vi "HandleObservationSync_003.vi"(8 "error in (no error)":errorcluster, 11 "S4GUI in":refnum<class "S4GUI.lvclass">) -> (0 "error out":errorcluster, 3 "S4GUI out":refnum<class "S4GUI.lvclass">)   [LabVIEW 2018, in "S4GUI.lvclass"] (continued)
          n222 = disable-structure shown="Enabled" {
            disable-tunnel: w542 -> [w576 w589]
            disable-tunnel: w541 -> [w575 w588]
            disable-tunnel: [w574 w589] -> w540
            disable-tunnel: [w573 w588] -> w539
            frame Disabled {
              n223 = call "Read WPROT.vi"("error in (no error)"=w575, "Instrument in"=w576) -> ("error out"=w579:errorcluster, "Opt_Selector.lvclass"=w580:refnum<class "Opt_Selector.lvclass">, "Instrument out"=w586:refnum<class "Instrument.lvclass">)  [unwired: 7 in]
              n224 = call-dynamic "Read State Machine.vi"("error in (no error)"=w579, "Device in"=w580) -> ("error out"=w582:errorcluster, "State Machine.lvclass"=w584:refnum<class "State Machine.lvclass">, "Device out"=w581:refnum<class "Opt_Selector.lvclass">)  [unwired: 7 in]
              n225 = call "Next State.vi"("error in (no error)"=w582, "New_State"=30, "State Machine in"=w584) -> ("error out"=w578:errorcluster, "State Machine out"=w577:refnum<class "State Machine.lvclass">)  [unwired: 7 in]
              n226 = call-dynamic "Write State Machine.vi"("error in (no error)"=w578, "State Machine.lvclass"=w577, "Device in"=w581) -> ("error out"=w585:errorcluster, "Device out"=w587:refnum<class "Opt_Selector.lvclass">)  [unwired: 7 in]
              n227 = call "Write WPROT.vi"("error in (no error)"=w585, "Opt_Selector.lvclass"=w587, "Instrument in"=w586) -> ("error out"=w573:errorcluster, "Instrument out"=w574:refnum<class "Instrument.lvclass">)  [unwired: 7 in]
            }
            frame Enabled {
              # "depois do homing no WPSEL, o homing do WPROT é feito automaticamente pelo ICS"
            }
          }
          n228 = call "Read ASEL.vi"("error in (no error)"=w539, "Instrument in"=w540) -> ("error out"=w556:errorcluster, "Opt_Selector.lvclass"=w557:refnum<class "Opt_Selector.lvclass">, "Instrument out"=w563:refnum<class "Instrument.lvclass">)  [unwired: 7 in]
          n229 = call-dynamic "Read State Machine.vi"("error in (no error)"=w556, "Device in"=w557) -> ("error out"=w559:errorcluster, "State Machine.lvclass"=w561:refnum<class "State Machine.lvclass">, "Device out"=w558:refnum<class "Opt_Selector.lvclass">)  [unwired: 7 in]
          n230 = call "Next State.vi"("error in (no error)"=w559, "New_State"=30, "State Machine in"=w561) -> ("error out"=w555:errorcluster, "State Machine out"=w554:refnum<class "State Machine.lvclass">)  [unwired: 7 in]
          n231 = call-dynamic "Write State Machine.vi"("error in (no error)"=w555, "State Machine.lvclass"=w554, "Device in"=w558) -> ("error out"=w562:errorcluster, "Device out"=w564:refnum<class "Opt_Selector.lvclass">)  [unwired: 7 in]
          n232 = Increment(x=w565) -> (x+1=w567:u32)
          n233 = call "Write ASEL.vi"("error in (no error)"=w562, "Opt_Selector.lvclass"=w564, "Instrument in"=w563) -> ("error out"=w537:errorcluster, "Instrument out"=w538:refnum<class "Instrument.lvclass">)  [unwired: 7 in]
          n234 = call "Read GMIR.vi"("error in (no error)"=w537, "Instrument in"=w538) -> ("error out"=w545:errorcluster, "Opt_Continuous.lvclass"=w546:refnum<class "Opt_Continuous.lvclass">, "Instrument out"=w552:refnum<class "Instrument.lvclass">)  [unwired: 7 in]
          n235 = call-dynamic "Read State Machine.vi"("error in (no error)"=w545, "Device in"=w546) -> ("error out"=w548:errorcluster, "State Machine.lvclass"=w550:refnum<class "State Machine.lvclass">, "Device out"=w547:refnum<class "Opt_Continuous.lvclass">)  [unwired: 7 in]
          n236 = call "Next State.vi"("error in (no error)"=w548, "New_State"=30, "State Machine in"=w550) -> ("error out"=w544:errorcluster, "State Machine out"=w543:refnum<class "State Machine.lvclass">)  [unwired: 7 in]
          n237 = call-dynamic "Write State Machine.vi"("error in (no error)"=w544, "State Machine.lvclass"=w543, "Device in"=w547) -> ("error out"=w551:errorcluster, "Device out"=w553:refnum<class "Opt_Continuous.lvclass">)  [unwired: 7 in]
          n238 = call "Write GMIR.vi"("error in (no error)"=w551, "Opt_Continuous.lvclass"=w553, "Instrument in"=w552) -> ("error out"=w536:errorcluster, "Instrument out"=w535:refnum<class "Instrument.lvclass">)  [unwired: 7 in]
          n239 = call "Write Instrument.lvclass.vi"("error in (no error)"=w536, "Instrument.lvclass"=w535, "S4ACS_GUI in"=w572) -> ("error out"=w569:errorcluster, "S4ACS_GUI out"=w568:refnum<class "S4GUI.lvclass">)  [unwired: 7 in]
          n240 = Bundle By Name(cluster=w568, "Obs_state"=w567) -> (w566:refnum<class "S4GUI.lvclass">)
        }
        frame 223 {
          # "Espera terminar o homing de WPROT,ASEL e GFOC\nantes de seguir para o próximo estado."
          n241 = call "Read Instrument.lvclass.vi"("error in (no error)"=w614, "S4ACS_GUI in"=w615) -> ("error out"=w600:errorcluster, "Instrument.lvclass"=w601:refnum<class "Instrument.lvclass">, "S4ACS_GUI out"=w609:refnum<class "S4GUI.lvclass">)  [unwired: 7 in]
          n242 = call "Read ASEL.vi"("error in (no error)"=w600, "Instrument in"=w601) -> ("error out"=w605:errorcluster, "Opt_Selector.lvclass"=w591:refnum<class "Opt_Selector.lvclass">)  [unwired: 7 in, 1 out]
          n243 = call "Read GMIR.vi"("error in (no error)"=w600, "Instrument in"=w601) -> ("error out"=w602:errorcluster, "Opt_Continuous.lvclass"=w590:refnum<class "Opt_Continuous.lvclass">)  [unwired: 7 in, 1 out]
          n244 = disable-structure shown="Enabled" {
            disable-tunnel: [w619 w625] -> w608
            disable-tunnel: w601 -> [w618 _]
            disable-tunnel: w600 -> [w617 w625]
            disable-tunnel: [w616 0 ("State")] -> w599
            frame Disabled {
              n245 = call "Read WPROT.vi"("error in (no error)"=w617, "Instrument in"=w618) -> ("error out"=w621:errorcluster, "Opt_Selector.lvclass"=w620:refnum<class "Opt_Selector.lvclass">)  [unwired: 7 in, 1 out]
              n246 = call-dynamic "Read State Machine.vi"("error in (no error)"=w621, "Device in"=w620) -> ("error out"=w622:errorcluster, "State Machine.lvclass"=w623:refnum<class "State Machine.lvclass">)  [unwired: 7 in, 1 out]
              n247 = call-dynamic "Read State.vi"("error in (no error)"=w622, "State Machine in"=w623) -> ("error out"=w619:errorcluster, "State"=w616:i32)  [unwired: 7 in, 1 out]
            }
            frame Enabled {
            }
          }
          n248 = call-dynamic "Read State Machine.vi"("error in (no error)"=w605, "Device in"=w591) -> ("error out"=w606:errorcluster, "State Machine.lvclass"=w607:refnum<class "State Machine.lvclass">)  [unwired: 7 in, 1 out]
          n249 = call-dynamic "Read State Machine.vi"("error in (no error)"=w602, "Device in"=w590) -> ("error out"=w603:errorcluster, "State Machine.lvclass"=w604:refnum<class "State Machine.lvclass">)  [unwired: 7 in, 1 out]
          n250 = Increment(x=w611) -> (x+1=w610:u32)
          n251 = call-dynamic "Read State.vi"("error in (no error)"=w606, "State Machine in"=w607) -> ("error out"=w594:errorcluster, "State"=w598:i32)  [unwired: 7 in, 1 out]
          n252 = call-dynamic "Read State.vi"("error in (no error)"=w603, "State Machine in"=w604) -> ("error out"=w593:errorcluster, "State"=w597:i32)  [unwired: 7 in, 1 out]
          n253 = Compound Arithmetic op=ADD(w599, w598, w597) -> (w596:i32)
          n254 = Equal To 0?(x=w596) -> (x = 0?=w595:bool)
          n255 = Merge Errors(w608, w594, w593) -> (w592:errorcluster)
          n256 = Select(t=w610, s=w595, f=w611) -> (s? t:f=w612:u32)
          n257 = Bundle By Name(cluster=w609, "Obs_state"=w612) -> (w613:refnum<class "S4GUI.lvclass">)
        }
        frame 224 {
          # "40 x 0.25 = 10s"
          # "40 x 0.25 = 10s"
          # "40 x 0.25 = 10s"
          # "Manda WPSEL para OFF, CALW para OFF e ASEL para OFF"
          n258 = call "Read Instrument.lvclass.vi"("error in (no error)"=w699, "S4ACS_GUI in"=w700) -> ("error out"=w685:errorcluster, "Instrument.lvclass"=w686:refnum<class "Instrument.lvclass">, "S4ACS_GUI out"=w701:refnum<class "S4GUI.lvclass">)  [unwired: 7 in]
          n259 = call "Read WPSEL.vi"("error in (no error)"=w685, "Instrument in"=w686) -> ("error out"=w681:errorcluster, "Opt_Selector.lvclass"=w680:refnum<class "Opt_Selector.lvclass">, "Instrument out"=w693:refnum<class "Instrument.lvclass">)  [unwired: 7 in]
          n260 = call "Write target.vi"("error in (no error)"=w681, "target"=80.0, "Optics in"=w680) -> ("error out"=w684:errorcluster, "Optics out"=w679:refnum<class "Opt_Selector.lvclass">)  [unwired: 7 in]
          n261 = call "Write target name.vi"("error in (no error)"=w684, "target name"="OFF", "Optics in"=w679) -> ("error out"=w677:errorcluster, "Optics out"=w678:refnum<class "Opt_Selector.lvclass">)  [unwired: 7 in]
          n262 = call-dynamic "Read State Machine.vi"("error in (no error)"=w677, "Device in"=w678) -> ("error out"=w688:errorcluster, "State Machine.lvclass"=w690:refnum<class "State Machine.lvclass">, "Device out"=w687:refnum<class "Opt_Selector.lvclass">)  [unwired: 7 in]
          n263 = call "Next State.vi"("error in (no error)"=w688, "New_State"=1, "State Machine in"=w690) -> ("error out"=w638:errorcluster, "State Machine out"=w640:refnum<class "State Machine.lvclass">)  [unwired: 7 in]
          n264 = call-dynamic "Write Timer.vi"("error in (no error)"=w638, "Timer"=u32 40, "State Machine in"=w640) -> ("error out"=w637:errorcluster, "State Machine out"=w639:refnum<class "State Machine.lvclass">)  [unwired: 7 in]
          n265 = call-dynamic "Write State Machine.vi"("error in (no error)"=w637, "State Machine.lvclass"=w639, "Device in"=w687) -> ("error out"=w692:errorcluster, "Device out"=w694:refnum<class "Opt_Selector.lvclass">)  [unwired: 7 in]
          n266 = Increment(x=w691) -> (x+1=w696:u32)
          n267 = call "Write WPSEL.vi"("error in (no error)"=w692, "Opt_Selector.lvclass"=w694, "Instrument in"=w693) -> ("error out"=w652:errorcluster, "Instrument out"=w651:refnum<class "Instrument.lvclass">)  [unwired: 7 in]
          n268 = call "Read CALW.vi"("error in (no error)"=w652, "Instrument in"=w651) -> ("error out"=w668:errorcluster, "Opt_Selector.lvclass"=w650:refnum<class "Opt_Selector.lvclass">, "Instrument out"=w648:refnum<class "Instrument.lvclass">)  [unwired: 7 in]
          n269 = call "Write target.vi"("error in (no error)"=w668, "target"=0.0, "Optics in"=w650) -> ("error out"=w671:errorcluster, "Optics out"=w667:refnum<class "Opt_Selector.lvclass">)  [unwired: 7 in]
          n270 = call "Write target name.vi"("error in (no error)"=w671, "target name"="OFF", "Optics in"=w667) -> ("error out"=w665:errorcluster, "Optics out"=w666:refnum<class "Opt_Selector.lvclass">)  [unwired: 7 in]
          n271 = call-dynamic "Read State Machine.vi"("error in (no error)"=w665, "Device in"=w666) -> ("error out"=w673:errorcluster, "State Machine.lvclass"=w675:refnum<class "State Machine.lvclass">, "Device out"=w672:refnum<class "Opt_Selector.lvclass">)  [unwired: 7 in]
          n272 = call "Next State.vi"("error in (no error)"=w673, "New_State"=1, "State Machine in"=w675) -> ("error out"=w634:errorcluster, "State Machine out"=w635:refnum<class "State Machine.lvclass">)  [unwired: 7 in]
          n273 = call-dynamic "Write Timer.vi"("error in (no error)"=w634, "Timer"=u32 40, "State Machine in"=w635) -> ("error out"=w633:errorcluster, "State Machine out"=w632:refnum<class "State Machine.lvclass">)  [unwired: 7 in]
          n274 = call-dynamic "Write State Machine.vi"("error in (no error)"=w633, "State Machine.lvclass"=w632, "Device in"=w672) -> ("error out"=w676:errorcluster, "Device out"=w649:refnum<class "Opt_Selector.lvclass">)  [unwired: 7 in]
          n275 = call "Write CALW.vi"("error in (no error)"=w676, "Opt_Selector.lvclass"=w649, "Instrument in"=w648) -> ("error out"=w647:errorcluster, "Instrument out"=w646:refnum<class "Instrument.lvclass">)  [unwired: 7 in]
          n276 = call "Read ASEL.vi"("error in (no error)"=w647, "Instrument in"=w646) -> ("error out"=w656:errorcluster, "Opt_Selector.lvclass"=w645:refnum<class "Opt_Selector.lvclass">, "Instrument out"=w643:refnum<class "Instrument.lvclass">)  [unwired: 7 in]
          n277 = call "Write target.vi"("error in (no error)"=w656, "target"=0.0, "Optics in"=w645) -> ("error out"=w659:errorcluster, "Optics out"=w655:refnum<class "Opt_Selector.lvclass">)  [unwired: 7 in]
          n278 = call "Write target name.vi"("error in (no error)"=w659, "target name"="OFF", "Optics in"=w655) -> ("error out"=w653:errorcluster, "Optics out"=w654:refnum<class "Opt_Selector.lvclass">)  [unwired: 7 in]
          n279 = call-dynamic "Read State Machine.vi"("error in (no error)"=w653, "Device in"=w654) -> ("error out"=w661:errorcluster, "State Machine.lvclass"=w663:refnum<class "State Machine.lvclass">, "Device out"=w660:refnum<class "Opt_Selector.lvclass">)  [unwired: 7 in]
          n280 = call "Next State.vi"("error in (no error)"=w661, "New_State"=1, "State Machine in"=w663) -> ("error out"=w628:errorcluster, "State Machine out"=w629:refnum<class "State Machine.lvclass">)  [unwired: 7 in]
          n281 = call-dynamic "Write Timer.vi"("error in (no error)"=w628, "Timer"=u32 40, "State Machine in"=w629) -> ("error out"=w627:errorcluster, "State Machine out"=w626:refnum<class "State Machine.lvclass">)  [unwired: 7 in]
          n282 = call-dynamic "Write State Machine.vi"("error in (no error)"=w627, "State Machine.lvclass"=w626, "Device in"=w660) -> ("error out"=w664:errorcluster, "Device out"=w644:refnum<class "Opt_Selector.lvclass">)  [unwired: 7 in]
          n283 = call "Write ASEL.vi"("error in (no error)"=w664, "Opt_Selector.lvclass"=w644, "Instrument in"=w643) -> ("error out"=w641:errorcluster, "Instrument out"=w642:refnum<class "Instrument.lvclass">)  [unwired: 7 in]
          n284 = call "Write Instrument.lvclass.vi"("error in (no error)"=w641, "Instrument.lvclass"=w642, "S4ACS_GUI in"=w701) -> ("error out"=w698:errorcluster, "S4ACS_GUI out"=w697:refnum<class "S4GUI.lvclass">)  [unwired: 7 in]
          n285 = Bundle By Name(cluster=w697, "Obs_state"=w696) -> (w695:refnum<class "S4GUI.lvclass">)
        }
        frame 225 {
          # "Espera terminar o movimento de WPSEL, ASEL e CALW para CLEAR."
          n286 = call "Read Instrument.lvclass.vi"("error in (no error)"=w730, "S4ACS_GUI in"=w731) -> ("error out"=w713:errorcluster, "Instrument.lvclass"=w714:refnum<class "Instrument.lvclass">, "S4ACS_GUI out"=w722:refnum<class "S4GUI.lvclass">)  [unwired: 7 in]
          n287 = call "Read ASEL.vi"("error in (no error)"=w713, "Instrument in"=w714) -> ("error out"=w718:errorcluster, "Opt_Selector.lvclass"=w704:refnum<class "Opt_Selector.lvclass">)  [unwired: 7 in, 1 out]
          n288 = call "Read CALW.vi"("error in (no error)"=w713, "Instrument in"=w714) -> ("error out"=w715:errorcluster, "Opt_Selector.lvclass"=w703:refnum<class "Opt_Selector.lvclass">)  [unwired: 7 in, 1 out]
          n289 = call "Read WPSEL.vi"("error in (no error)"=w713, "Instrument in"=w714) -> ("error out"=w727:errorcluster, "Opt_Selector.lvclass"=w726:refnum<class "Opt_Selector.lvclass">)  [unwired: 7 in, 1 out]
          n290 = call-dynamic "Read State Machine.vi"("error in (no error)"=w715, "Device in"=w703) -> ("error out"=w716:errorcluster, "State Machine.lvclass"=w717:refnum<class "State Machine.lvclass">)  [unwired: 7 in, 1 out]
          n291 = call-dynamic "Read State Machine.vi"("error in (no error)"=w718, "Device in"=w704) -> ("error out"=w719:errorcluster, "State Machine.lvclass"=w720:refnum<class "State Machine.lvclass">)  [unwired: 7 in, 1 out]
          n292 = call-dynamic "Read State Machine.vi"("error in (no error)"=w727, "Device in"=w726) -> ("error out"=w728:errorcluster, "State Machine.lvclass"=w729:refnum<class "State Machine.lvclass">)  [unwired: 7 in, 1 out]
          n293 = call-dynamic "Read State.vi"("error in (no error)"=w719, "State Machine in"=w720) -> ("error out"=w707:errorcluster, "State"=w711:i32)  [unwired: 7 in, 1 out]
          n294 = call-dynamic "Read State.vi"("error in (no error)"=w716, "State Machine in"=w717) -> ("error out"=w706:errorcluster, "State"=w710:i32)  [unwired: 7 in, 1 out]
          n295 = call-dynamic "Read State.vi"("error in (no error)"=w728, "State Machine in"=w729) -> ("error out"=w721:errorcluster, "State"=w712:i32)  [unwired: 7 in, 1 out]
          n296 = Compound Arithmetic op=ADD(w712, w711, w710) -> (w709:i32)
          n297 = Equal To 0?(x=w709) -> (x = 0?=w708:bool)
          n298 = Merge Errors(w721, w707, w706) -> (w705:errorcluster)
          n299 = Select(t=u32 0, s=w708, f=w723) -> (s? t:f=w724:u32)
          n300 = Bundle By Name(cluster=w722, "Obs_state"=w724) -> (w725:refnum<class "S4GUI.lvclass">)
        }
        frame 230 {
          # "PARK:\nWPSEL = OFF\n(WPROT=NA)\nCALW=SHUTTER\nASEL=OFF"
          n301 = call "Read Instrument.lvclass.vi"("error in (no error)"=w800, "S4ACS_GUI in"=w801) -> ("error out"=w793:errorcluster, "Instrument.lvclass"=w794:refnum<class "Instrument.lvclass">, "S4ACS_GUI out"=w735:refnum<class "S4GUI.lvclass">)  [unwired: 7 in]
          n302 = call "Read WPSEL.vi"("error in (no error)"=w793, "Instrument in"=w794) -> ("error out"=w756:errorcluster, "Opt_Selector.lvclass"=w759:refnum<class "Opt_Selector.lvclass">, "Instrument out"=w789:refnum<class "Instrument.lvclass">)  [unwired: 7 in]
          n303 = call "Write target name.vi"("error in (no error)"=w756, "target name"="OFF", "Optics in"=w759) -> ("error out"=w755:errorcluster, "Optics out"=w758:refnum<class "Opt_Selector.lvclass">)  [unwired: 7 in]
          n304 = call "Write target.vi"("error in (no error)"=w755, "target"=80.0, "Optics in"=w758) -> ("error out"=w754:errorcluster, "Optics out"=w757:refnum<class "Opt_Selector.lvclass">)  [unwired: 7 in]
          n305 = call-dynamic "Read State Machine.vi"("error in (no error)"=w754, "Device in"=w757) -> ("error out"=w785:errorcluster, "State Machine.lvclass"=w787:refnum<class "State Machine.lvclass">, "Device out"=w784:refnum<class "Opt_Selector.lvclass">)  [unwired: 7 in]
          n306 = call "Next State.vi"("error in (no error)"=w785, "New_State"=1, "State Machine in"=w787) -> ("error out"=w764:errorcluster, "State Machine out"=w765:refnum<class "State Machine.lvclass">)  [unwired: 7 in]
          n307 = call-dynamic "Write State Machine.vi"("error in (no error)"=w764, "State Machine.lvclass"=w765, "Device in"=w784) -> ("error out"=w788:errorcluster, "Device out"=w790:refnum<class "Opt_Selector.lvclass">)  [unwired: 7 in]
          n308 = Increment(x=w795) -> (x+1=w797:u32)
          n309 = call "Write WPSEL.vi"("error in (no error)"=w788, "Opt_Selector.lvclass"=w790, "Instrument in"=w789) -> ("error out"=w768:errorcluster, "Instrument out"=w769:refnum<class "Instrument.lvclass">)  [unwired: 7 in]
          n310 = call "Read CALW.vi"("error in (no error)"=w768, "Instrument in"=w769) -> ("error out"=w748:errorcluster, "Opt_Selector.lvclass"=w747:refnum<class "Opt_Selector.lvclass">, "Instrument out"=w782:refnum<class "Instrument.lvclass">)  [unwired: 7 in]
          n311 = call "Write target name.vi"("error in (no error)"=w748, "target name"="SHUTTER", "Optics in"=w747) -> ("error out"=w751:errorcluster, "Optics out"=w746:refnum<class "Opt_Selector.lvclass">)  [unwired: 7 in]
          n312 = call "Write target.vi"("error in (no error)"=w751, "target"=216.0, "Optics in"=w746) -> ("error out"=w744:errorcluster, "Optics out"=w745:refnum<class "Opt_Selector.lvclass">)  [unwired: 7 in]
          n313 = call-dynamic "Read State Machine.vi"("error in (no error)"=w744, "Device in"=w745) -> ("error out"=w778:errorcluster, "State Machine.lvclass"=w780:refnum<class "State Machine.lvclass">, "Device out"=w777:refnum<class "Opt_Selector.lvclass">)  [unwired: 7 in]
          n314 = call "Next State.vi"("error in (no error)"=w778, "New_State"=1, "State Machine in"=w780) -> ("error out"=w762:errorcluster, "State Machine out"=w763:refnum<class "State Machine.lvclass">)  [unwired: 7 in]
          n315 = call-dynamic "Write State Machine.vi"("error in (no error)"=w762, "State Machine.lvclass"=w763, "Device in"=w777) -> ("error out"=w781:errorcluster, "Device out"=w783:refnum<class "Opt_Selector.lvclass">)  [unwired: 7 in]
          n316 = call "Write CALW.vi"("error in (no error)"=w781, "Opt_Selector.lvclass"=w783, "Instrument in"=w782) -> ("error out"=w766:errorcluster, "Instrument out"=w767:refnum<class "Instrument.lvclass">)  [unwired: 7 in]
          n317 = call "Read ASEL.vi"("error in (no error)"=w766, "Instrument in"=w767) -> ("error out"=w737:errorcluster, "Opt_Selector.lvclass"=w740:refnum<class "Opt_Selector.lvclass">, "Instrument out"=w775:refnum<class "Instrument.lvclass">)  [unwired: 7 in]
          n318 = call "Write target name.vi"("error in (no error)"=w737, "target name"="OFF", "Optics in"=w740) -> ("error out"=w743:errorcluster, "Optics out"=w739:refnum<class "Opt_Selector.lvclass">)  [unwired: 7 in]
          n319 = call "Write target.vi"("error in (no error)"=w743, "target"=0.0, "Optics in"=w739) -> ("error out"=w736:errorcluster, "Optics out"=w738:refnum<class "Opt_Selector.lvclass">)  [unwired: 7 in]
          n320 = call-dynamic "Read State Machine.vi"("error in (no error)"=w736, "Device in"=w738) -> ("error out"=w771:errorcluster, "State Machine.lvclass"=w773:refnum<class "State Machine.lvclass">, "Device out"=w770:refnum<class "Opt_Selector.lvclass">)  [unwired: 7 in]
          n321 = call "Next State.vi"("error in (no error)"=w771, "New_State"=1, "State Machine in"=w773) -> ("error out"=w760:errorcluster, "State Machine out"=w761:refnum<class "State Machine.lvclass">)  [unwired: 7 in]
          n322 = call-dynamic "Write State Machine.vi"("error in (no error)"=w760, "State Machine.lvclass"=w761, "Device in"=w770) -> ("error out"=w774:errorcluster, "Device out"=w776:refnum<class "Opt_Selector.lvclass">)  [unwired: 7 in]
          n323 = call "Write ASEL.vi"("error in (no error)"=w774, "Opt_Selector.lvclass"=w776, "Instrument in"=w775) -> ("error out"=w792:errorcluster, "Instrument out"=w791:refnum<class "Instrument.lvclass">)  [unwired: 7 in]
          n324 = Tick Count (ms)() -> (millisecond timer value=w732:u32)
          n325 = local write "time1"(w732) -> ()
          n326 = Bundle By Name(cluster=w735, "Error Msg"="Parking in progress. Wait....") -> (w734:refnum<class "S4GUI.lvclass">)
          n327 = call "Write Instrument.lvclass.vi"("error in (no error)"=w792, "Instrument.lvclass"=w791, "S4ACS_GUI in"=w734) -> ("error out"=w799:errorcluster, "S4ACS_GUI out"=w798:refnum<class "S4GUI.lvclass">)  [unwired: 7 in]
          n328 = Bundle By Name(cluster=w798, "Obs_state"=w797) -> (w796:refnum<class "S4GUI.lvclass">)
        }
        frame 231 {
          # "Espera terminar o parking de WPSEL,CALW e ASEL\nantes de encerrar aplicacao (exit=True)."
          n329 = call "Read Instrument.lvclass.vi"("error in (no error)"=w837, "S4ACS_GUI in"=w838) -> ("error out"=w821:errorcluster, "Instrument.lvclass"=w822:refnum<class "Instrument.lvclass">, "S4ACS_GUI out"=w830:refnum<class "S4GUI.lvclass">)  [unwired: 7 in]
          n330 = call "Read CALW.vi"("error in (no error)"=w821, "Instrument in"=w822) -> ("error out"=w826:errorcluster, "Opt_Selector.lvclass"=w812:refnum<class "Opt_Selector.lvclass">)  [unwired: 7 in, 1 out]
          n331 = call "Read ASEL.vi"("error in (no error)"=w821, "Instrument in"=w822) -> ("error out"=w823:errorcluster, "Opt_Selector.lvclass"=w811:refnum<class "Opt_Selector.lvclass">)  [unwired: 7 in, 1 out]
          n332 = call "Read WPSEL.vi"("error in (no error)"=w821, "Instrument in"=w822) -> ("error out"=w834:errorcluster, "Opt_Selector.lvclass"=w833:refnum<class "Opt_Selector.lvclass">)  [unwired: 7 in, 1 out]
          n333 = call-dynamic "Read State Machine.vi"("error in (no error)"=w826, "Device in"=w812) -> ("error out"=w827:errorcluster, "State Machine.lvclass"=w828:refnum<class "State Machine.lvclass">)  [unwired: 7 in, 1 out]
          n334 = call-dynamic "Read State Machine.vi"("error in (no error)"=w823, "Device in"=w811) -> ("error out"=w824:errorcluster, "State Machine.lvclass"=w825:refnum<class "State Machine.lvclass">)  [unwired: 7 in, 1 out]
          n335 = call-dynamic "Read State Machine.vi"("error in (no error)"=w834, "Device in"=w833) -> ("error out"=w835:errorcluster, "State Machine.lvclass"=w836:refnum<class "State Machine.lvclass">)  [unwired: 7 in, 1 out]
          n336 = Increment(x=w804) -> (x+1=w831:u32)
          n337 = call-dynamic "Read State.vi"("error in (no error)"=w827, "State Machine in"=w828) -> ("error out"=w815:errorcluster, "State"=w819:i32)  [unwired: 7 in, 1 out]
          n338 = call-dynamic "Read State.vi"("error in (no error)"=w824, "State Machine in"=w825) -> ("error out"=w814:errorcluster, "State"=w818:i32)  [unwired: 7 in, 1 out]
          n339 = call-dynamic "Read State.vi"("error in (no error)"=w835, "State Machine in"=w836) -> ("error out"=w829:errorcluster, "State"=w820:i32)  [unwired: 7 in, 1 out]
          n340 = Compound Arithmetic op=ADD(w820, w819, w818) -> (w817:i32)
          n341 = Equal To 0?(x=w817) -> (x = 0?=w816:bool)
          n342 = Merge Errors(w829, w815, w814) -> (w813:errorcluster)
          n343 = Select(t=w831, s=w816, f=w804) -> (s? t:f=w803:u32)
          n344 = Tick Count (ms)() -> (millisecond timer value=w810:u32)
          n345 = local read "time1"() -> (w808:u32)
          n346 = Subtract(x=w810, y=w808) -> (x-y=w809:u32)
          n347 = To Double Precision Float(number=w809) -> (double precision float=w807:dbl)
          n348 = Greater?(x=w807, y=30000.0) -> (0:w805:bool)
          n349 = case shown="True" w805 {
            tunnel: w804 -> [_ w841]
            tunnel: [w839 w840] -> w802
            tunnel: w803 -> [w839 _]
            frame False {
            }
            frame True {
              n350 = Increment(x=w841) -> (x+1=w840:u32)
            }
          }
          n351 = Bundle By Name(cluster=w830, "Obs_state"=w802) -> (w832:refnum<class "S4GUI.lvclass">)
        }
        frame 232 {
          n352 = Increment(x=w843) -> (x+1=w842:u32)
          n353 = Tick Count (ms)() -> (millisecond timer value=w844:u32)
          n354 = local write "time1"(w844) -> ()
          n355 = Bundle By Name(cluster=w847, "Obs_state"=w842) -> (w845:refnum<class "S4GUI.lvclass">)
        }
        frame 233 {
          # "Aguarda 1s para atualização do painel da GUI antes de encerrar..."
          n356 = local read "time1"() -> (w851:u32)
          n357 = Tick Count (ms)() -> (millisecond timer value=w852:u32)
          n358 = Subtract(x=w852, y=w851) -> (x-y=w850:u32)
          n359 = Greater?(x=w850, y=u32 1000) -> (0:w848:bool)
          n360 = case shown="True" w848 {
            tunnel: w854 -> [w858 w860]
            tunnel: [w858 w859] -> w853
            frame False {
            }
            frame True {
              n361 = Increment(x=w860) -> (x+1=w859:u32)
            }
          }
          n362 = Bundle By Name(cluster=w857, "Obs_state"=w853) -> (w855:refnum<class "S4GUI.lvclass">)
        }
        frame 234 {
          n363 = Bundle By Name(cluster=w865, "Obs_state"=u32 0, "exit"=TRUE) -> (w863:refnum<class "S4GUI.lvclass">)
        }
        frame 251 {
          n364 = flat-sequence {
            tunnel: w914 -> [w1069]
            tunnel: [w1069] -> w913
            frame #0 {
              n365 = Tick Count (ms)() -> (millisecond timer value=→"time3":u32)
            }
          }
          n366 = call-dynamic "Read AcquisitionA.vi"("error in (no error)"=w913, "S4ACS_GUI in"=w931) -> ("error out"=w898:errorcluster, "Acquisition.lvclass"=w896:refnum<class "Acquisition.lvclass">, "S4ACS_GUI out"=w933:refnum<class "S4GUI.lvclass">)  [unwired: 7 in]
          n367 = call-dynamic "Read enabled.vi"("error in (no error)"=w898, "Server in"=w896) -> ("error out"=w897:errorcluster, "enabled"=w893:bool, "Server out"=w895:refnum<class "Acquisition.lvclass">)  [unwired: 7 in]
          n368 = call "Read connection.vi"("error in (no error)"=w897, "Server in"=w895) -> ("error out"=w929:errorcluster, "connection"=w899:bool, "Server out"=w928:refnum<class "Acquisition.lvclass">)  [unwired: 7 in]
          n369 = And(x=w899, y=w893) -> (x .and. y?=w894:bool)
          n370 = case shown="True" w894 {
            tunnel: [w1049 w1068] -> w934
            tunnel: [w1048 w1067] -> w932
            tunnel: w929 -> [w1048 w1066]
            tunnel: w928 -> [w1049 w1065]
            tunnel: w893 -> [w1045 _]
            tunnel: [w1044 u32 0] -> w892
            frame False {
              n371 = Select(t=u32 1, s=w1045, f=u32 0) -> (s? t:f=w1044:u32)
            }
            frame True {
              # "configura o canal,\nmas não dispara\na exposicao."
              n372 = call-dynamic "Read Channel.vi"("error in (no error)"=w1066, "Acquisition in"=w1065) -> ("error out"=w1055:errorcluster, "Channel.lvclass"=w1057:refnum<class "Channel.lvclass">, "Acquisition out"=w1064:refnum<class "Acquisition.lvclass">)  [unwired: 7 in]
              n373 = call-dynamic "Write expose.vi"("error in (no error)"=w1055, "expose"=FALSE, "Channel in"=w1057) -> ("error out"=w1054:errorcluster, "Channel out"=w1056:refnum<class "Channel.lvclass">)  [unwired: 7 in]
              n374 = call-dynamic "Read State Machine.vi"("error in (no error)"=w1054, "Device in"=w1056) -> ("error out"=w1061:errorcluster, "State Machine.lvclass"=w1063:refnum<class "State Machine.lvclass">, "Device out"=w1059:refnum<class "Channel.lvclass">)  [unwired: 7 in]
              n375 = call "Next State.vi"("error in (no error)"=w1061, "New_State"=1, "State Machine in"=w1063) -> ("error out"=w1051:errorcluster, "State Machine out"=w1052:refnum<class "State Machine.lvclass">)  [unwired: 7 in]
              n376 = call-dynamic "Write State Machine.vi"("error in (no error)"=w1051, "State Machine.lvclass"=w1052, "Device in"=w1059) -> ("error out"=w1058:errorcluster, "Device out"=w1060:refnum<class "Channel.lvclass">)  [unwired: 7 in]
              n377 = call-dynamic "Write Channel.vi"("error in (no error)"=w1058, "Channel.lvclass"=w1060, "Acquisition in"=w1064) -> ("error out"=w1067:errorcluster, "Acquisition out"=w1068:refnum<class "Acquisition.lvclass">)  [unwired: 7 in]
            }
          }
          n378 = call-dynamic "Write AcquisitionA.vi"("error in (no error)"=w932, "Acquisition.lvclass"=w934, "S4ACS_GUI in"=w933) -> ("error out"=w924:errorcluster, "S4ACS_GUI out"=w923:refnum<class "S4GUI.lvclass">)  [unwired: 7 in]
          n379 = call "Read AcquisitionB.vi"("error in (no error)"=w924, "S4ACS_GUI in"=w923) -> ("error out"=w882:errorcluster, "Acquisition.lvclass"=w884:refnum<class "Acquisition.lvclass">, "S4ACS_GUI out"=w925:refnum<class "S4GUI.lvclass">)  [unwired: 7 in]
          n380 = call-dynamic "Read enabled.vi"("error in (no error)"=w882, "Server in"=w884) -> ("error out"=w881:errorcluster, "enabled"=w866:bool, "Server out"=w883:refnum<class "Acquisition.lvclass">)  [unwired: 7 in]
          n381 = call "Read connection.vi"("error in (no error)"=w881, "Server in"=w883) -> ("error out"=w910:errorcluster, "connection"=w885:bool, "Server out"=w911:refnum<class "Acquisition.lvclass">)  [unwired: 7 in]
          n382 = And(x=w885, y=w866) -> (x .and. y?=w886:bool)
          n383 = case shown="True" w886 {
            tunnel: [w1024 w1043] -> w909
            tunnel: [w1023 w1042] -> w908
            tunnel: w910 -> [w1023 w1041]
            tunnel: w911 -> [w1024 w1040]
            tunnel: [w1020 u32 0 ("f")] -> w889
            tunnel: w866 -> [w1019 _]
            frame False {
              n384 = Select(t=u32 2, s=w1019, f=u32 0) -> (s? t:f=w1020:u32)
            }
            frame True {
              # "configura o canal,\nmas não dispara\na exposicao."
              n385 = call-dynamic "Read Channel.vi"("error in (no error)"=w1041, "Acquisition in"=w1040) -> ("error out"=w1030:errorcluster, "Channel.lvclass"=w1032:refnum<class "Channel.lvclass">, "Acquisition out"=w1039:refnum<class "Acquisition.lvclass">)  [unwired: 7 in]
              n386 = call-dynamic "Write expose.vi"("error in (no error)"=w1030, "expose"=FALSE, "Channel in"=w1032) -> ("error out"=w1029:errorcluster, "Channel out"=w1031:refnum<class "Channel.lvclass">)  [unwired: 7 in]
              n387 = call-dynamic "Read State Machine.vi"("error in (no error)"=w1029, "Device in"=w1031) -> ("error out"=w1036:errorcluster, "State Machine.lvclass"=w1038:refnum<class "State Machine.lvclass">, "Device out"=w1034:refnum<class "Channel.lvclass">)  [unwired: 7 in]
              n388 = call "Next State.vi"("error in (no error)"=w1036, "New_State"=1, "State Machine in"=w1038) -> ("error out"=w1026:errorcluster, "State Machine out"=w1027:refnum<class "State Machine.lvclass">)  [unwired: 7 in]
              n389 = call-dynamic "Write State Machine.vi"("error in (no error)"=w1026, "State Machine.lvclass"=w1027, "Device in"=w1034) -> ("error out"=w1033:errorcluster, "Device out"=w1035:refnum<class "Channel.lvclass">)  [unwired: 7 in]
              n390 = call-dynamic "Write Channel.vi"("error in (no error)"=w1033, "Channel.lvclass"=w1035, "Acquisition in"=w1039) -> ("error out"=w1042:errorcluster, "Acquisition out"=w1043:refnum<class "Acquisition.lvclass">)  [unwired: 7 in]
            }
          }
          n391 = call "Write AcquisitionB.vi"("error in (no error)"=w908, "Acquisition.lvclass"=w909, "S4ACS_GUI in"=w925) -> ("error out"=w920:errorcluster, "S4ACS_GUI out"=w919:refnum<class "S4GUI.lvclass">)  [unwired: 7 in]
          n392 = call-dynamic "Read AcquisitionC.vi"("error in (no error)"=w920, "S4ACS_GUI in"=w919) -> ("error out"=w878:errorcluster, "Acquisition.lvclass"=w880:refnum<class "Acquisition.lvclass">, "S4ACS_GUI out"=w922:refnum<class "S4GUI.lvclass">)  [unwired: 7 in]
          n393 = call-dynamic "Read enabled.vi"("error in (no error)"=w878, "Server in"=w880) -> ("error out"=w877:errorcluster, "enabled"=w867:bool, "Server out"=w879:refnum<class "Acquisition.lvclass">)  [unwired: 7 in]
          n394 = call "Read connection.vi"("error in (no error)"=w877, "Server in"=w879) -> ("error out"=w906:errorcluster, "connection"=w876:bool, "Server out"=w907:refnum<class "Acquisition.lvclass">)  [unwired: 7 in]
          n395 = And(x=w876, y=w867) -> (x .and. y?=w875:bool)
          n396 = case shown="True" w875 {
            tunnel: [w999 w1018] -> w905
            tunnel: [w998 w1017] -> w904
            tunnel: w906 -> [w998 w1016]
            tunnel: w907 -> [w999 w1015]
            tunnel: [w995 u32 0 ("f")] -> w888
            tunnel: w867 -> [w994 _]
            frame False {
              n397 = Select(t=u32 4, s=w994, f=u32 0) -> (s? t:f=w995:u32)
            }
            frame True {
              # "configura o canal,\nmas não dispara\na exposicao."
              n398 = call-dynamic "Read Channel.vi"("error in (no error)"=w1016, "Acquisition in"=w1015) -> ("error out"=w1005:errorcluster, "Channel.lvclass"=w1007:refnum<class "Channel.lvclass">, "Acquisition out"=w1014:refnum<class "Acquisition.lvclass">)  [unwired: 7 in]
              n399 = call-dynamic "Write expose.vi"("error in (no error)"=w1005, "expose"=FALSE, "Channel in"=w1007) -> ("error out"=w1004:errorcluster, "Channel out"=w1006:refnum<class "Channel.lvclass">)  [unwired: 7 in]
              n400 = call-dynamic "Read State Machine.vi"("error in (no error)"=w1004, "Device in"=w1006) -> ("error out"=w1011:errorcluster, "State Machine.lvclass"=w1013:refnum<class "State Machine.lvclass">, "Device out"=w1009:refnum<class "Channel.lvclass">)  [unwired: 7 in]
              n401 = call "Next State.vi"("error in (no error)"=w1011, "New_State"=1, "State Machine in"=w1013) -> ("error out"=w1001:errorcluster, "State Machine out"=w1002:refnum<class "State Machine.lvclass">)  [unwired: 7 in]
              n402 = call-dynamic "Write State Machine.vi"("error in (no error)"=w1001, "State Machine.lvclass"=w1002, "Device in"=w1009) -> ("error out"=w1008:errorcluster, "Device out"=w1010:refnum<class "Channel.lvclass">)  [unwired: 7 in]
              n403 = call-dynamic "Write Channel.vi"("error in (no error)"=w1008, "Channel.lvclass"=w1010, "Acquisition in"=w1014) -> ("error out"=w1017:errorcluster, "Acquisition out"=w1018:refnum<class "Acquisition.lvclass">)  [unwired: 7 in]
            }
          }
          n404 = call-dynamic "Write AcquisitionC.vi"("error in (no error)"=w904, "Acquisition.lvclass"=w905, "S4ACS_GUI in"=w922) -> ("error out"=w918:errorcluster, "S4ACS_GUI out"=w917:refnum<class "S4GUI.lvclass">)  [unwired: 7 in]
          n405 = call-dynamic "Read AcquisitionD.vi"("error in (no error)"=w918, "S4ACS_GUI in"=w917) -> ("error out"=w872:errorcluster, "Acquisition.lvclass"=w874:refnum<class "Acquisition.lvclass">, "S4ACS_GUI out"=w921:refnum<class "S4GUI.lvclass">)  [unwired: 7 in]
          n406 = call-dynamic "Read enabled.vi"("error in (no error)"=w872, "Server in"=w874) -> ("error out"=w871:errorcluster, "enabled"=w868:bool, "Server out"=w873:refnum<class "Acquisition.lvclass">)  [unwired: 7 in]
          n407 = call "Read connection.vi"("error in (no error)"=w871, "Server in"=w873) -> ("error out"=w902:errorcluster, "connection"=w870:bool, "Server out"=w903:refnum<class "Acquisition.lvclass">)  [unwired: 7 in]
          n408 = And(x=w870, y=w868) -> (x .and. y?=w869:bool)
          n409 = case shown="True" w869 {
            tunnel: [w974 w993] -> w901
            tunnel: [w973 w992] -> w900
            tunnel: w902 -> [w973 w991]
            tunnel: w903 -> [w974 w990]
            tunnel: [w970 u32 0 ("f")] -> w887
            tunnel: w868 -> [w969 _]
            frame False {
              n410 = Select(t=u32 8, s=w969, f=u32 0) -> (s? t:f=w970:u32)
            }
            frame True {
              # "configura o canal,\nmas não dispara\na exposicao."
              n411 = call-dynamic "Read Channel.vi"("error in (no error)"=w991, "Acquisition in"=w990) -> ("error out"=w980:errorcluster, "Channel.lvclass"=w982:refnum<class "Channel.lvclass">, "Acquisition out"=w989:refnum<class "Acquisition.lvclass">)  [unwired: 7 in]
              n412 = call-dynamic "Write expose.vi"("error in (no error)"=w980, "expose"=FALSE, "Channel in"=w982) -> ("error out"=w979:errorcluster, "Channel out"=w981:refnum<class "Channel.lvclass">)  [unwired: 7 in]
              n413 = call-dynamic "Read State Machine.vi"("error in (no error)"=w979, "Device in"=w981) -> ("error out"=w986:errorcluster, "State Machine.lvclass"=w988:refnum<class "State Machine.lvclass">, "Device out"=w984:refnum<class "Channel.lvclass">)  [unwired: 7 in]
              n414 = call "Next State.vi"("error in (no error)"=w986, "New_State"=1, "State Machine in"=w988) -> ("error out"=w976:errorcluster, "State Machine out"=w977:refnum<class "State Machine.lvclass">)  [unwired: 7 in]
              n415 = call-dynamic "Write State Machine.vi"("error in (no error)"=w976, "State Machine.lvclass"=w977, "Device in"=w984) -> ("error out"=w983:errorcluster, "Device out"=w985:refnum<class "Channel.lvclass">)  [unwired: 7 in]
              n416 = call-dynamic "Write Channel.vi"("error in (no error)"=w983, "Channel.lvclass"=w985, "Acquisition in"=w989) -> ("error out"=w992:errorcluster, "Acquisition out"=w993:refnum<class "Acquisition.lvclass">)  [unwired: 7 in]
            }
          }
          n417 = call-dynamic "Write AcquisitionD.vi"("error in (no error)"=w900, "Acquisition.lvclass"=w901, "S4ACS_GUI in"=w921) -> ("error out"=w916:errorcluster, "S4ACS_GUI out"=w915:refnum<class "S4GUI.lvclass">)  [unwired: 7 in]
          n418 = Compound Arithmetic op=ADD(w892, w889, w888, w887) -> (w891:u32)
          n419 = case shown="0, Default" w891 {
            tunnel: w927 -> [w938 _ _ _ _ _ _ _ _ _ _ _ _ _ _ _]
            tunnel: [w937 u32 1 ("Obs_state") u32 1 ("Obs_state") u32 1 ("Obs_state") u32 1 ("Obs_state") u32 1 ("Obs_state") u32 1 ("Obs_state") u32 1 ("Obs_state") u32 1 ("Obs_state") u32 1 ("Obs_state") u32 1 ("Obs_state") u32 1 ("Obs_state") u32 1 ("Obs_state") u32 1 ("Obs_state") u32 1 ("Obs_state") u32 1 ("Obs_state")] -> w926
            tunnel: ["" ("Error Msg") "ERROR: Lost channel 1 connection... - HandleObservationSync.vi state 251" ("Error Msg") "ERROR: Lost channel 2 connection...- HandleObservationSync.vi state 251" ("Error Msg") "ERROR: Lost channels 1 and 2 connection...- HandleObservationSync.vi state 251" ("Error Msg") "ERROR: Lost channel 3 connection...- HandleObservationSync.vi state 251" ("Error Msg") "ERROR: Lost channels 1 and  3 connection...- HandleObservationSync.vi state 251" ("Error Msg") "ERROR:  Lost channels 2 and  3 connection...- HandleObservationSync.vi state 251" ("Error Msg") "ERROR:  Lost channels 1, 2 and  3 connection...- HandleObservationSync.vi state 251" ("Error Msg") "ERROR: Lost channel 4 connection...- HandleObservationSync.vi state 251" ("Error Msg") "ERROR:  Lost channels 1 and 4 connection...- HandleObservationSync.vi state 251" ("Error Msg") "ERROR:  Lost channels 2 and 4 connection...- HandleObservationSync.vi state 251" ("Error Msg") "ERROR: Lost channels 1, 2 and 4 connection...- HandleObservationSync.vi state 251" ("Error Msg") "ERROR: Lost channels 3 and 4 connection...- HandleObservationSync.vi state 251" ("Error Msg") "ERROR: Lost channels 1, 3 and 4 connection...- HandleObservationSync.vi state 251" ("Error Msg") "ERROR: Lost channels 2, 3 and 4 connection...- HandleObservationSync.vi state 251" ("Error Msg") "ERROR: Lost channels 1, 2, 3 and 4 connection...- HandleObservationSync.vi state 251" ("Error Msg")] -> w890
            frame 0, Default {
              n420 = Tick Count (ms)() -> (millisecond timer value=→"time307":u32)
              n421 = Increment(x=w938) -> (x+1=w937:u32)
            }
            frame 1 {
            }
            frame 2 {
            }
            frame 3 {
            }
            frame 4 {
            }
            frame 5 {
            }
            frame 6 {
            }
            frame 7 {
            }
            frame 8 {
            }
            frame 9 {
            }
            frame 10 {
            }
            frame 11 {
            }
            frame 12 {
            }
            frame 13 {
            }
            frame 14 {
            }
            frame 15 {
            }
          }
          n422 = Bundle By Name(cluster=w915, "Obs_state"=w926, "cyclesDone"=u32 0, "Error Msg"=w890) -> (w930:refnum<class "S4GUI.lvclass">)
        }
        frame 252 {
          w1092 = 38 ("x")
          w1095 = 28 ("x")
          # "Se algum canal foi pra 38: Texp inválido \npara a configuração do CCD."
          # "Se algum canal foi pra 28: ERRO na inicialização."
          # "Espera terminar a execução da preparação\ndos 4 canais antes de ir ao proximo passo \nda Observação."
          n423 = flat-sequence {
            tunnel: w1124 -> [w1261]
            tunnel: [w1261] -> w1123
            frame #0 {
              n424 = Tick Count (ms)() -> (millisecond timer value=→"time4":u32)
            }
          }
          n425 = call-dynamic "Read AcquisitionA.vi"("error in (no error)"=w1123, "S4ACS_GUI in"=w1133) -> ("error out"=w1121:errorcluster, "Acquisition.lvclass"=w1122:refnum<class "Acquisition.lvclass">, "S4ACS_GUI out"=w1135:refnum<class "S4GUI.lvclass">)  [unwired: 7 in]
          n426 = call "Read connection.vi"("error in (no error)"=w1121, "Server in"=w1122) -> ("error out"=w1119:errorcluster, "connection"=w1118:bool, "Server out"=w1120:refnum<class "Acquisition.lvclass">)  [unwired: 7 in]
          n427 = case shown="True" w1118 {
            tunnel: w1120 -> [w1244 w1260]
            tunnel: w1119 -> [w1243 w1259]
            tunnel: [w1244 w1257] -> w1136
            tunnel: [w1243 w1256] -> w1134
            tunnel: [0 ("State") w1246] -> w1091
            frame False {
            }
            frame True {
              n428 = call-dynamic "Read Channel.vi"("error in (no error)"=w1259, "Acquisition in"=w1260) -> ("error out"=w1255:errorcluster, "Channel.lvclass"=w1254:refnum<class "Channel.lvclass">, "Acquisition out"=w1258:refnum<class "Acquisition.lvclass">)  [unwired: 7 in]
              n429 = call-dynamic "Read State Machine.vi"("error in (no error)"=w1255, "Device in"=w1254) -> ("error out"=w1248:errorcluster, "State Machine.lvclass"=w1250:refnum<class "State Machine.lvclass">, "Device out"=w1252:refnum<class "Channel.lvclass">)  [unwired: 7 in]
              n430 = call-dynamic "Read State.vi"("error in (no error)"=w1248, "State Machine in"=w1250) -> ("error out"=w1247:errorcluster, "State"=w1246:i32, "State Machine out"=w1249:refnum<class "State Machine.lvclass">)  [unwired: 7 in]
              n431 = call-dynamic "Write State Machine.vi"("error in (no error)"=w1247, "State Machine.lvclass"=w1249, "Device in"=w1252) -> ("error out"=w1251:errorcluster, "Device out"=w1253:refnum<class "Channel.lvclass">)  [unwired: 7 in]
              n432 = call-dynamic "Write Channel.vi"("error in (no error)"=w1251, "Channel.lvclass"=w1253, "Acquisition in"=w1258) -> ("error out"=w1256:errorcluster, "Acquisition out"=w1257:refnum<class "Acquisition.lvclass">)  [unwired: 7 in]
            }
          }
          n433 = call-dynamic "Write AcquisitionA.vi"("error in (no error)"=w1134, "Acquisition.lvclass"=w1136, "S4ACS_GUI in"=w1135) -> ("error out"=w1130:errorcluster, "S4ACS_GUI out"=w1129:refnum<class "S4GUI.lvclass">)  [unwired: 7 in]
          n434 = call "Read AcquisitionB.vi"("error in (no error)"=w1130, "S4ACS_GUI in"=w1129) -> ("error out"=w1113:errorcluster, "Acquisition.lvclass"=w1116:refnum<class "Acquisition.lvclass">, "S4ACS_GUI out"=w1117:refnum<class "S4GUI.lvclass">)  [unwired: 7 in]
          n435 = call "Read connection.vi"("error in (no error)"=w1113, "Server in"=w1116) -> ("error out"=w1112:errorcluster, "connection"=w1114:bool, "Server out"=w1115:refnum<class "Acquisition.lvclass">)  [unwired: 7 in]
          n436 = case shown="True" w1114 {
            tunnel: w1115 -> [w1226 w1242]
            tunnel: w1112 -> [w1225 w1241]
            tunnel: [w1226 w1239] -> w1111
            tunnel: [w1225 w1238] -> w1110
            tunnel: [0 ("State") w1228] -> w1090
            frame False {
            }
            frame True {
              n437 = call-dynamic "Read Channel.vi"("error in (no error)"=w1241, "Acquisition in"=w1242) -> ("error out"=w1237:errorcluster, "Channel.lvclass"=w1236:refnum<class "Channel.lvclass">, "Acquisition out"=w1240:refnum<class "Acquisition.lvclass">)  [unwired: 7 in]
              n438 = call-dynamic "Read State Machine.vi"("error in (no error)"=w1237, "Device in"=w1236) -> ("error out"=w1230:errorcluster, "State Machine.lvclass"=w1232:refnum<class "State Machine.lvclass">, "Device out"=w1234:refnum<class "Channel.lvclass">)  [unwired: 7 in]
              n439 = call-dynamic "Read State.vi"("error in (no error)"=w1230, "State Machine in"=w1232) -> ("error out"=w1229:errorcluster, "State"=w1228:i32, "State Machine out"=w1231:refnum<class "State Machine.lvclass">)  [unwired: 7 in]
              n440 = call-dynamic "Write State Machine.vi"("error in (no error)"=w1229, "State Machine.lvclass"=w1231, "Device in"=w1234) -> ("error out"=w1233:errorcluster, "Device out"=w1235:refnum<class "Channel.lvclass">)  [unwired: 7 in]
              n441 = call-dynamic "Write Channel.vi"("error in (no error)"=w1233, "Channel.lvclass"=w1235, "Acquisition in"=w1240) -> ("error out"=w1238:errorcluster, "Acquisition out"=w1239:refnum<class "Acquisition.lvclass">)  [unwired: 7 in]
            }
          }
          n442 = call "Write AcquisitionB.vi"("error in (no error)"=w1110, "Acquisition.lvclass"=w1111, "S4ACS_GUI in"=w1117) -> ("error out"=w1128:errorcluster, "S4ACS_GUI out"=w1127:refnum<class "S4GUI.lvclass">)  [unwired: 7 in]
          n443 = call-dynamic "Read AcquisitionC.vi"("error in (no error)"=w1128, "S4ACS_GUI in"=w1127) -> ("error out"=w1108:errorcluster, "Acquisition.lvclass"=w1109:refnum<class "Acquisition.lvclass">, "S4ACS_GUI out"=w1132:refnum<class "S4GUI.lvclass">)  [unwired: 7 in]
          n444 = call "Read connection.vi"("error in (no error)"=w1108, "Server in"=w1109) -> ("error out"=w1107:errorcluster, "connection"=w1105:bool, "Server out"=w1106:refnum<class "Acquisition.lvclass">)  [unwired: 7 in]
          n445 = case shown="True" w1105 {
            tunnel: w1106 -> [w1208 w1224]
            tunnel: w1107 -> [w1207 w1223]
            tunnel: [w1208 w1221] -> w1104
            tunnel: [w1207 w1220] -> w1103
            tunnel: [0 ("State") w1210] -> w1089
            frame False {
            }
            frame True {
              n446 = call-dynamic "Read Channel.vi"("error in (no error)"=w1223, "Acquisition in"=w1224) -> ("error out"=w1219:errorcluster, "Channel.lvclass"=w1218:refnum<class "Channel.lvclass">, "Acquisition out"=w1222:refnum<class "Acquisition.lvclass">)  [unwired: 7 in]
              n447 = call-dynamic "Read State Machine.vi"("error in (no error)"=w1219, "Device in"=w1218) -> ("error out"=w1212:errorcluster, "State Machine.lvclass"=w1214:refnum<class "State Machine.lvclass">, "Device out"=w1216:refnum<class "Channel.lvclass">)  [unwired: 7 in]
              n448 = call-dynamic "Read State.vi"("error in (no error)"=w1212, "State Machine in"=w1214) -> ("error out"=w1211:errorcluster, "State"=w1210:i32, "State Machine out"=w1213:refnum<class "State Machine.lvclass">)  [unwired: 7 in]
              n449 = call-dynamic "Write State Machine.vi"("error in (no error)"=w1211, "State Machine.lvclass"=w1213, "Device in"=w1216) -> ("error out"=w1215:errorcluster, "Device out"=w1217:refnum<class "Channel.lvclass">)  [unwired: 7 in]
              n450 = call-dynamic "Write Channel.vi"("error in (no error)"=w1215, "Channel.lvclass"=w1217, "Acquisition in"=w1222) -> ("error out"=w1220:errorcluster, "Acquisition out"=w1221:refnum<class "Acquisition.lvclass">)  [unwired: 7 in]
            }
          }
          n451 = call-dynamic "Write AcquisitionC.vi"("error in (no error)"=w1103, "Acquisition.lvclass"=w1104, "S4ACS_GUI in"=w1132) -> ("error out"=w1126:errorcluster, "S4ACS_GUI out"=w1125:refnum<class "S4GUI.lvclass">)  [unwired: 7 in]
          n452 = call-dynamic "Read AcquisitionD.vi"("error in (no error)"=w1126, "S4ACS_GUI in"=w1125) -> ("error out"=w1100:errorcluster, "Acquisition.lvclass"=w1102:refnum<class "Acquisition.lvclass">, "S4ACS_GUI out"=w1131:refnum<class "S4GUI.lvclass">)  [unwired: 7 in]
          n453 = call "Read connection.vi"("error in (no error)"=w1100, "Server in"=w1102) -> ("error out"=w1099:errorcluster, "connection"=w1098:bool, "Server out"=w1101:refnum<class "Acquisition.lvclass">)  [unwired: 7 in]
          n454 = case shown="True" w1098 {
            tunnel: w1101 -> [w1190 w1206]
            tunnel: w1099 -> [w1189 w1205]
            tunnel: [w1190 w1203] -> w1097
            tunnel: [w1189 w1202] -> w1096
            tunnel: [0 ("State") w1192] -> w1088
            frame False {
            }
            frame True {
              n455 = call-dynamic "Read Channel.vi"("error in (no error)"=w1205, "Acquisition in"=w1206) -> ("error out"=w1201:errorcluster, "Channel.lvclass"=w1200:refnum<class "Channel.lvclass">, "Acquisition out"=w1204:refnum<class "Acquisition.lvclass">)  [unwired: 7 in]
              n456 = call-dynamic "Read State Machine.vi"("error in (no error)"=w1201, "Device in"=w1200) -> ("error out"=w1194:errorcluster, "State Machine.lvclass"=w1196:refnum<class "State Machine.lvclass">, "Device out"=w1198:refnum<class "Channel.lvclass">)  [unwired: 7 in]
              n457 = call-dynamic "Read State.vi"("error in (no error)"=w1194, "State Machine in"=w1196) -> ("error out"=w1193:errorcluster, "State"=w1192:i32, "State Machine out"=w1195:refnum<class "State Machine.lvclass">)  [unwired: 7 in]
              n458 = call-dynamic "Write State Machine.vi"("error in (no error)"=w1193, "State Machine.lvclass"=w1195, "Device in"=w1198) -> ("error out"=w1197:errorcluster, "Device out"=w1199:refnum<class "Channel.lvclass">)  [unwired: 7 in]
              n459 = call-dynamic "Write Channel.vi"("error in (no error)"=w1197, "Channel.lvclass"=w1199, "Acquisition in"=w1204) -> ("error out"=w1202:errorcluster, "Acquisition out"=w1203:refnum<class "Acquisition.lvclass">)  [unwired: 7 in]
            }
          }
          n460 = call-dynamic "Write AcquisitionD.vi"("error in (no error)"=w1096, "Acquisition.lvclass"=w1097, "S4ACS_GUI in"=w1131) -> ("error out"=w1082:errorcluster, "S4ACS_GUI out"=w1083:refnum<class "S4GUI.lvclass">)  [unwired: 7 in]
          n461 = Equal?(x=w1092, y=w1091) -> (x = y?=w1078:bool)
          n462 = Equal?(x=w1095, y=w1091) -> (x = y?=w1073:bool)
          n463 = Equal?(x=w1092, y=w1090) -> (x = y?=w1072:bool)
          n464 = Equal?(x=w1095, y=w1090) -> (x = y?=w1074:bool)
          n465 = Equal?(x=w1092, y=w1089) -> (x = y?=w1071:bool)
          n466 = Equal?(x=w1095, y=w1089) -> (x = y?=w1075:bool)
          n467 = Equal?(x=w1092, y=w1088) -> (x = y?=w1077:bool)
          n468 = Equal?(x=w1095, y=w1088) -> (x = y?=w1076:bool)
          n469 = call-dynamic "VerifyAcqIdle.vi"("error in (no error)"=w1082, "S4GUI in"=w1083) -> ("error out"=w1080:errorcluster, "idle"=w1079:bool, "S4GUI out"=w1081:refnum<class "S4GUI.lvclass">)  [unwired: 7 in]
          n470 = Compound Arithmetic op=OR(w1073, w1074, w1075, w1076) -> (w1087:bool)
          n471 = Compound Arithmetic op=OR(w1078, w1072, w1071, w1077) -> (w1086:bool)
          n472 = Build Array(w1087, w1086) -> (w1085:bool[])
          n473 = Boolean Array To Number(Boolean array=w1085) -> (number=w1084:u32)
          n474 = case shown="2" w1084 {
            tunnel: w1081 -> [w1146 w1171 w1184 w1188]
            tunnel: [w1145 w1170 w1183 w1187] -> w1093
            tunnel: w1094 -> [w1147 _ _ _]
            tunnel: w1079 -> [w1143 _ _ _]
            tunnel: w1078 -> [_ _ w1181 _]
            tunnel: w1072 -> [_ _ w1180 _]
            tunnel: w1071 -> [_ _ w1179 _]
            tunnel: w1077 -> [_ _ w1178 _]
            tunnel: w1076 -> [_ w1163 _ _]
            tunnel: w1075 -> [_ w1164 _ _]
            tunnel: w1074 -> [_ w1165 _ _]
            tunnel: w1073 -> [_ w1166 _ _]
            frame 0, Default {
              n475 = local read "time307"() -> (w1141:u32)
              n476 = Tick Count (ms)() -> (millisecond timer value=w1142:u32)
              n477 = Subtract(x=w1142, y=w1141) -> (x-y=w1140:u32)
              n478 = Greater?(x=w1140, y=u32 10000) -> (0:w1138:bool)
              n479 = case shown="False" w1138 {
                tunnel: w1147 -> [w1151 _]
                tunnel: [w1150 u32 1 ("Obs_state")] -> w1144
                tunnel: w1143 -> [w1149 _]
                tunnel: ["" w1156] -> w1137
                frame False {
                  n480 = disable-structure shown="Enabled" {
                    disable-tunnel: [299 ("t") 300] -> w1152
                    frame Disabled {
                    }
                    frame Enabled {
                    }
                  }
                  n481 = Select(t=w1152, s=w1149, f=w1151) -> (s? t:f=w1150:u32)
                }
                frame True {
                  n482 = Concatenate Strings("CHANNEL ERROR " ("string"), ": Not idle. S4GUI:HandleObservationSync.vi state 252." ("Error Msg")) -> (w1156:string)
                }
              }
              n483 = Bundle By Name(cluster=w1146, "Obs_state"=w1144, "Error Msg"=w1137) -> (w1145:refnum<class "S4GUI.lvclass">)
            }
            frame 1 {
              n484 = Build Array(w1166, w1165, w1164, w1163) -> (w1168:bool[])
              n485 = Boolean Array To Number(Boolean array=w1168) -> (number=w1167:u32)
              n486 = Number To Decimal String(number=w1167) -> (decimal integer string=w1161:string)  [unwired: 1 in]
              n487 = Concatenate Strings("CHANNEL ERROR < " ("string"), w1161, ">: Initialization failed. S4GUI:HandleObservationSync.vi state 252." ("Error Msg")) -> (w1160:string)
              n488 = Bundle By Name(cluster=w1171, "Obs_state"=u32 1, "Error Msg"=w1160) -> (w1170:refnum<class "S4GUI.lvclass">)
            }
            frame 2 {
              n489 = Build Array(w1181, w1180, w1179, w1178) -> (w1177:bool[])
              n490 = Boolean Array To Number(Boolean array=w1177) -> (number=w1173:u32)
              n491 = Number To Decimal String(number=w1173) -> (decimal integer string=w1172:string)  [unwired: 1 in]
              n492 = Concatenate Strings("CHANNEL ERROR < " ("string"), w1172, ">:  Invalid Exposition Time. S4GUI:HandleObservationSync.vi state 252." ("Error Msg")) -> (w1175:string)
              n493 = Bundle By Name(cluster=w1184, "Obs_state"=u32 1, "Error Msg"=w1175) -> (w1183:refnum<class "S4GUI.lvclass">)
            }
            frame 3 {
              n494 = Bundle By Name(cluster=w1188, "Obs_state"=u32 1, "Error Msg"="ERROR: Invalid configuration in the channels. S4GUI:HandleObservationSync.vi state 252.") -> (w1187:refnum<class "S4GUI.lvclass">)
            }
          }
        }
        frame 253 {
          # "Sem SyncBox, \ntrigger mode = 0 (internal)\nCom SyncBox\ntrigger mode = 6 (ext. start)"
          n495 = call-dynamic "Read Sync Box.lvclass.vi"("error in (no error)"=w1300, "SPARC4_AC in"=w1299) -> ("error out"=w1302:errorcluster, "Sync Box.lvclass"=w1303:refnum<class "Sync Box.lvclass">, "SPARC4_AC out"=w1298:refnum<class "S4GUI.lvclass">)  [unwired: 7 in]
          n496 = call "Read connection.vi"("error in (no error)"=w1302, "Server in"=w1303) -> ("error out"=w1301:errorcluster, "connection"=w1263:bool)  [unwired: 7 in, 1 out]
          n497 = case shown="True" w1263 {
            tunnel: [u8 6 ("TRIGGER_MODE") u8 0 ("TRIGGER_MODE")] -> w1280
            frame True {
            }
            frame False {
            }
          }
          n498 = call-dynamic "Read AcquisitionA.vi"("error in (no error)"=w1301, "S4ACS_GUI in"=w1298) -> ("error out"=w1285:errorcluster, "Acquisition.lvclass"=w1286:refnum<class "Acquisition.lvclass">, "S4ACS_GUI out"=w1284:refnum<class "S4GUI.lvclass">)  [unwired: 7 in]
